vi "Get Order Spectrum.vi"(6 "window type":T3(ring)=enum."Hanning", 7 "dB On (T)":bool=TRUE, 9 "pulse/revolution (1)":dbl=1.0 format="%.2f", 10 "speed profile":T2 {"speed [RPM]" format="%.2f"; "time [s]" format="%.2f"}, 11 "scaled signal [EU]":waveform(dbl)={"t0"=timestamp(0 s since 1904-01-01), "dt"=0.0, "Y"=[]}) -> (0 "average speed [rpm]":dbl format="%.2f", 1 "unit label":string, 3 "order spectrum":T1 {"order 0" format="%.2p"; "delta order" format="%.2p"; "magnitude" format="%.2f"})   [LabVIEW 2017]
doc: "Computes the order spectrum as power versus orders from <B>scaled signal</B>."
uses:
  <vilib>/addons/Sound and Vibration/Order Analysis/Tach Process/SubVIs/speed profile.ctl
  <vilib>/Analysis/baseanly.llb/Mean (DBL).vi
  <vilib>/Analysis/0measdsp.llb/Scaled Time Domain Window (DBL).vi
  <vilib>/Analysis/NI_AALPro.lvlib
  <vilib>/Analysis/NI_AALBase.lvlib
  <vilib>/addons/Sound and Vibration/Order Analysis/Tach Process/SoundVib_TachProcess.lvlib
panel:
  in  "average on speed?":bool
  # "Get Order Spectrum"
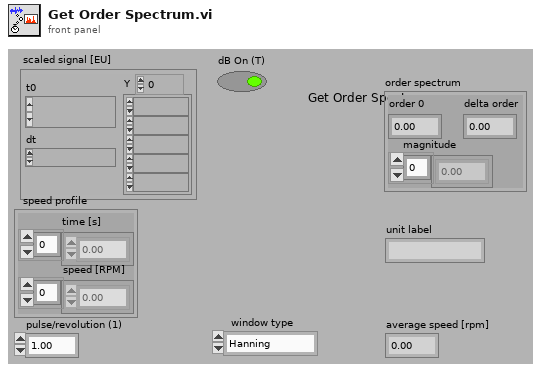
[diagram p1: front panel]
types:
  T1 = cluster{"order 0":dbl, "delta order":dbl, "magnitude":dbl[]}
  T2 = typedef "SoundVib_TachProcess.lvlib/speed profile.ctl" = cluster{"time [s]":dbl[], "speed [RPM]":dbl[]}
  T3 = enum16{"None ", "Hanning", "Hamming", "Blackman-Harris", "Exact Blackman", "Blackman", "Flat Top", "4 Term B-Harris ", "7 Term B-Harris", "Low Sidelobe"}
  T4 = typedef "svl_Channel Info.ctl" = cluster{"sensor sensitivity [mV/EU]":dbl, "engineering units":T5, "dB reference [EU]":dbl, "custom label":string, "weighting filter":T6, "pregain [dB]":dbl}
  T5 = typedef "svl_Engineering Units Text Ring.ctl" = u16
  T6 = typedef "svl_Weighting Filter Text Ring.ctl" = u16
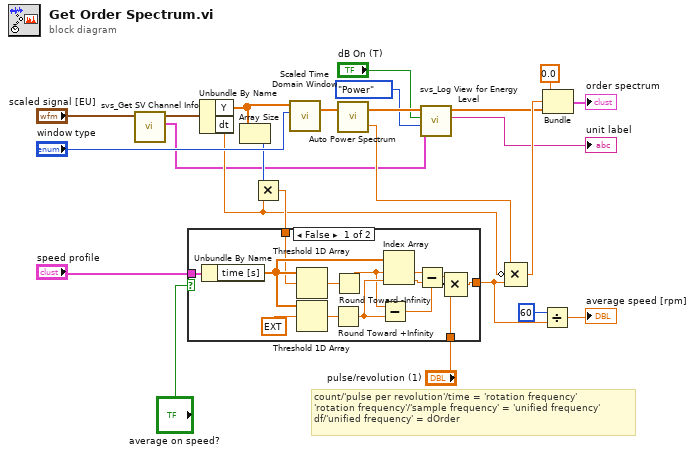
[diagram p0: block diagram]
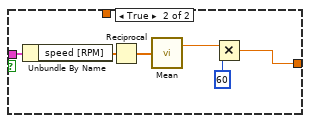
[diagram p2: hidden frame]
diagram:
  # "count/'pulse per revolution'/time = 'rotation frequency'\n'rotation frequency'/'sample frequency' = 'unified frequency'\ndf/'unified frequency' = dOrder"
  n1 = call <vilib>:"svs_Get SV Channel Info.vi"("scaled signal [EU]"="scaled signal [EU]") -> ("channel info"=w3:T4, "dup scaled signal [EU]"=w7:waveform(dbl))  [unwired: 8 in, 1 out]
  n2 = Unbundle By Name(w7) -> ("Y"=w13:dbl[], "dt"=w12:dbl)
  n3 = Array Size(array=w13) -> (size(s)=w20:i32)
  n4 = Multiply(x=w20, y=w12) -> (x*y=w19:dbl)
  n5 = case shown="False" "average on speed?" {
    tunnel: "speed profile" -> [w36 w43]
    tunnel: w19 -> [w30 _]
    tunnel: [w28 w40] -> w15
    tunnel: "pulse/revolution (1)" -> [w25 _]
    frame False {
      n6 = Unbundle By Name(w36) -> ("time [s]"=w33:dbl[])
      n7 = Threshold 1D Array(2:w30, 3:w33) -> (0:w35:dbl)  [unwired: 1 in]
      n8 = Threshold 1D Array(2:ext 0.0 ("fractional index or x"), 3:w33) -> (0:w34:dbl)  [unwired: 1 in]
      n9 = Round Toward +Infinity(x=w34) -> (ceil(x): smallest int >= x=w32:dbl)
      n10 = Round Toward -Infinity(1:w35) -> (0:w31:dbl)
      n11 = Subtract(x=w31, y=w32) -> (x-y=w26:dbl)
      n12 = Index Array(array=w33, index #1=w31, index #2=w32) -> (element #1=w38:dbl, element #2=w37:dbl)
      n13 = Subtract(x=w38, y=w37) -> (x-y=w27:dbl)
      n14 = Compound Arithmetic op=MULTIPLY(w27, invert w26, w25) -> (w28:dbl)
    }
    frame True {
      n15 = Unbundle By Name(w43) -> ("speed [RPM]"=w42:dbl[])
      n16 = Reciprocal(x=w42) -> (1/x=w44:dbl[])
      n17 = call-poly <vilib>:"Mean.vi"("X"=w44) -> ("mean"=w41:dbl)  [unwired: 1 out]
      n18 = Multiply(x=w41, y=60) -> (x*y=w40:dbl)
    }
  }
  n19 = call-poly <vilib>:"Scaled Time Domain Window.vi"("window"="window type", "X"=w13) -> ("Windowed X"=w23:dbl[])  [unwired: 7 in, 2 out]
  n20 = call <vilib>:"Auto Power Spectrum.vi"("Signal (V)"=w23) -> ("df"=w22:dbl, "Power Spectrum (V^2 rms)"=w6:dbl[])  [unwired: 1 in]
  n21 = call <vilib>:"svs_Log View for Energy Level.vi"("channel info"=w3, "view mode"=enum16{"Power", "Amplitude"}."Power", "dB On (T)"="dB On (T)", "energy level [EU^2 rms]"=w6) -> ("unit label"=→"unit label":string, "log view [dB EU]"=w2:dbl[])  [unwired: 6 in]
  n22 = Compound Arithmetic op=MULTIPLY(w22, invert w12, w15) -> (w11:dbl)
  n23 = Divide(x=60, y=w15) -> (x/y=→"average speed [rpm]":dbl)
  n24 = Bundle(0.0, w11, "log view [dB EU]"=w2) -> (→"order spectrum":cluster{dbl, dbl, "log view [dB EU]":dbl[]})  [unwired: 1 in]
